vi "LAKESHORE_11_01_2023_R_VS_T_DEMO_3.vi"() -> ()   [LabVIEW 2020]
panel:
  out "Filename":string
  in  "Total iterations":i32
  out "Temperature":dbl
  in  "Average Number of readings \nper iterations":i32
  in  "Save data":bool
  out "Resistance":dbl
  in  "Channel":T1(ring)
  out "XY Graph":cluster{"X":dbl[], "Y":dbl[]}[](graph)
  in  "VISA resource name":refnum<visa-resource-name>
  # "LAKE SHORE 372"
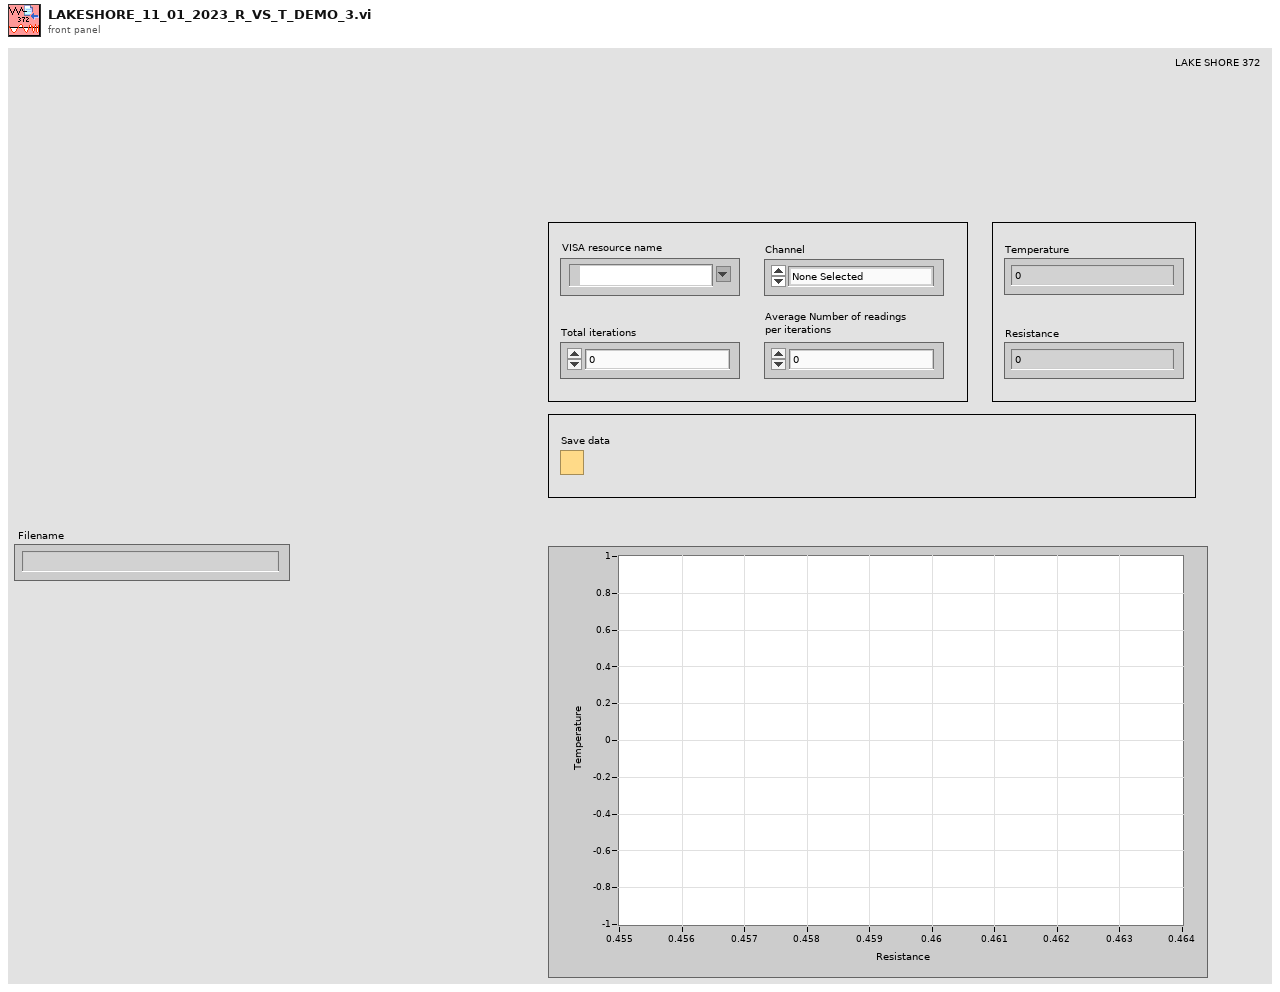
[diagram p1: front panel]
types:
  T1 = enum16{"None Selected", "1", "2", "3", "4", "5", "6", "7", "8", "9", "10", "11", "12", "13", "14", "15", "16"}
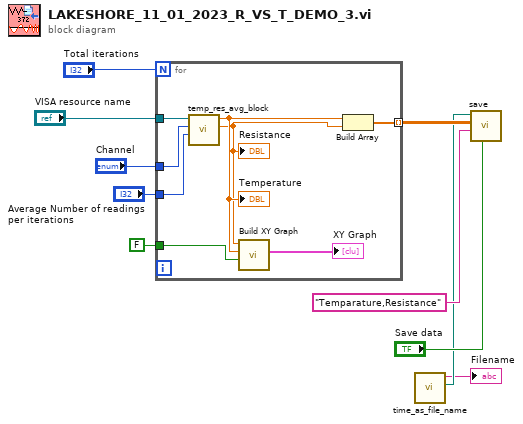
[diagram p0: block diagram]
diagram:
  n1 = for {
    N: "Total iterations" -> [_]
    tunnel: "VISA resource name" -> [w16]
    tunnel: FALSE ("Reset") -> [w17]
    tunnel: "Channel" -> [w15]
    tunnel: "Average Number of readings \nper iterations" -> [w14]
    tunnel: [w11] -> w3 mode=indexing
    n2 = call "temp_res_avg_block.vi"("Avg"=w14, "Channel in"=w15, "VISA Refnum in"=w16) -> ("Numeric"=w12:dbl, "Numeric 2"=w13:dbl)  [unwired: 7 in]
    "Resistance" <- w12
    "Temperature" <- w13
    n3 = call "Build XY Graph"("Reset"=w17, "Y Input"=w13, "X Input"=w12) -> ("XY Graph"=→"XY Graph":cluster{"X":dbl[], "Y":dbl[]}[])  [unwired: 7 in, 1 out]
    n4 = Build Array(w13, w12) -> (w11:dbl[])
  }
  n5 = call "time_as_file_name.vi"() -> ("Path"=w2:path, "Filename"=→"Filename":string)  [unwired: 10 in]
  n6 = call "save.vi"("Save data"="Save data", "String"="Temparature,Resistance", "Array"=w3, "File_name"=w2) -> ()  [unwired: 8 in]
